vi "BC Schedule and Data Update.vi"() -> ()   [LabVIEW 2019]
doc: "This example program configures Card Number 0 as a Bus Controller\nto transmit a schedule of three messages. The schedule is\ncreated in such a way that the messages are transmitted at\nfrequencies of 100Hz, 50Hz and 25Hz (or every 10ms, 20ms and\n40ms, respectively).\n\nThe program watches the 'HIT' bit associated with the 0843H\nBC->RT message. When the message is transmitted and the\nbit is set, the program updates the data words."
uses:
  <instrlib>/BTICardLib/Private/Initialize By Card Number and Core Number.vi
  <instrlib>/BTI1553Lib/Private/Channel/Configure/Configure Channel From XML.vi
  <instrlib>/BTICardLib/BTICardLV.lvlib
  <instrlib>/BTI1553Lib/BTI1553LV.lvlib
panel:
  out "core number":i32
  out "channel number":i32
  out "Data":u16[](array[numeric]) format="%04x"
  in  "Configuration Filename":string="BCScheduleDataUpdate.FINF"
  in  "stop":bool
  out "error out":errorcluster
  in  "Card Number":i32
  # "LabVIEW RT"
  # "Mil-Std-1553: BC Schedule and Data Update"
  # "©2016 Astronics Ballard Technology"
  # "This example program configures Card Number 0 as a Bus Controller\nto transmit a schedule of three messages. The schedule is\ncreated in such a way that the messages are transmitted at\nfrequencies of 100Hz, 50Hz and 25Hz (or every 10ms, 20ms and\n40ms, respectively).\n\nThe program watches the 'HIT' bit associated with the 0843H\nBC->RT message. When the message is transmitted and the\nbit is set, the program updates the data words."
  # "LabVIEW RT can parse both XML and Binary (FINF or Fast Infoset) configuration files. While the Binary files are non-human readable, they can be loaded and parsed much more quickly than XML and are also smaller. These can also be used in LabVIEW for Windows.\n\nLabVIEW RT examples use the Binary configuration file and the corollary \"Configure From Bin\" VIs. Using the XML is as simple as switching the polymorphic configuration VI from \"Binary\" to \"XML\" and changing the Configuration Filename above."
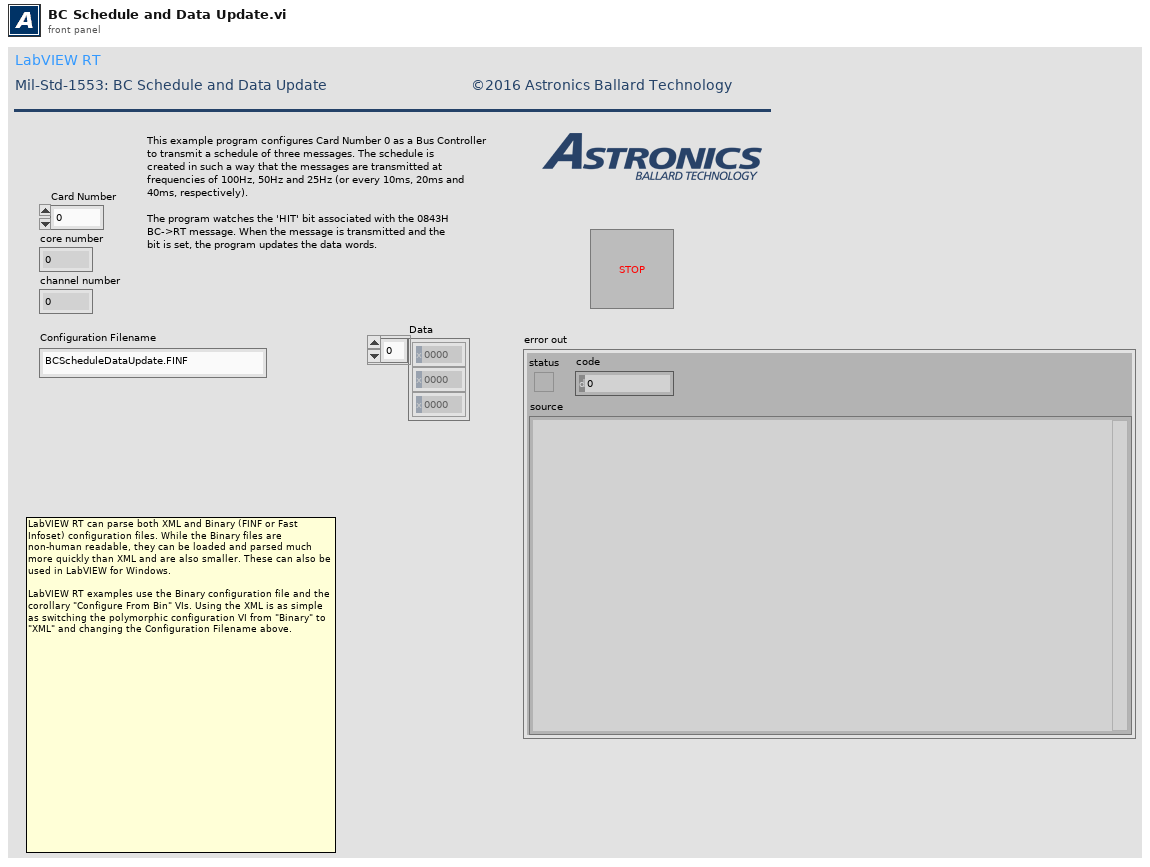
[diagram p1: front panel]
types:
  T1 = typedef "BTI1553LV.lvlib/1553 Message Fields.ctl" = cluster{"msgflag":u16, "msgopt":u16, "anyerror":bool, "noresponse":bool, "allretriesfailed":bool, "protocolerror":bool, "wrongsyncerror":bool, "datacounterror":bool, "manchestererror":bool, "parityerror":bool, "worderror":bool, "systemerror":bool, "hit":bool, "reserved":u8, "channelnumber":i32, "transmittedcwd1":bool, "transmittedcwd2":bool, "transmittedswd1":bool, "transmittedswd2":bool, "receivedcwd1":bool, "receivedcwd2":bool, "receivedswd1":bool, "receivedswd2":bool, "transmitteddwd":bool, "receiveddwd":bool, "reserved":i8, "reserved":i8, "bus":u32, "resptime1":u16, "resptime2":u16, "datacount":u16, "extflag":u16, "timetagh":u32, "timetag_hitcount":u32, "elapsetime_mintime_maxtime":u32, "cwd1":u16, "cwd2":u16, "swd1":u16, "swd2":u16, "data":u16[], "extra":u16[]}
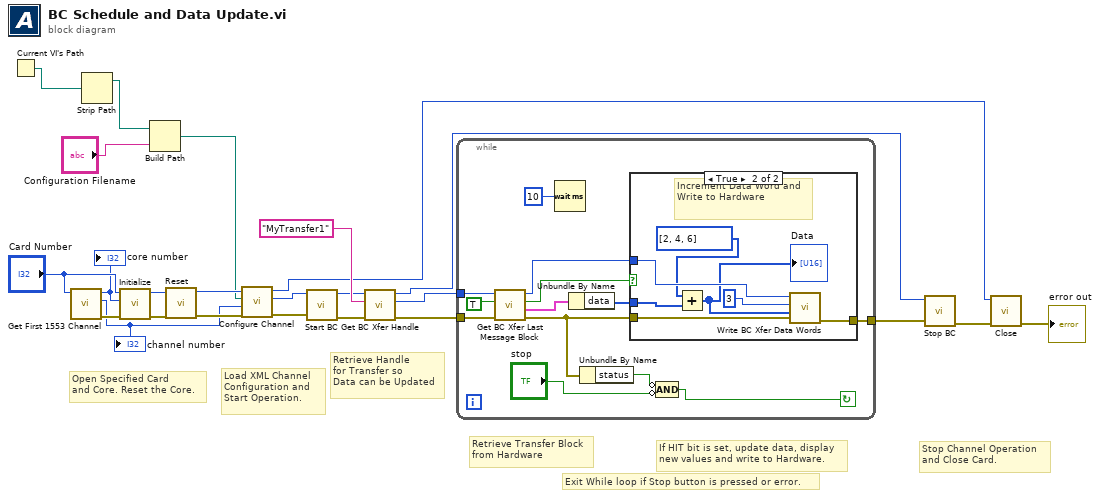
[diagram p0: block diagram]
diagram:
  # "Stop Channel Operation\nand Close Card."
  # "Exit While loop if Stop button is pressed or error."
  # "If HIT bit is set, update data, display\nnew values and write to Hardware."
  # "Retrieve Transfer Block\nfrom Hardware"
  # "Retrieve Handle\nfor Transfer so\nData can be Updated"
  # "Load XML Channel\nConfiguration and \nStart Operation."
  # "Open Specified Card\nand Core. Reset the Core."
  n1 = Current VI's Path() -> (path=w14:path)
  n2 = call "Get First 1553 Channel.vi"("Card Number"="Card Number") -> ("error out"=w4:errorcluster, "Channel Number"=w1:i32, "Core Number"=w2:i32)  [unwired: 8 in]
  "channel number" <- w1
  "core number" <- w2
  n3 = Strip Path(path=w14) -> (stripped path=w16:path)  [unwired: 1 out]
  n4 = call-poly <instrlib>:"Initialize.vi"("error in (no error)"=w4, "core number"=w2, "card number"="Card Number") -> ("error out"=w24:errorcluster, "core handle out"=w23:u64)  [unwired: 7 in]
  n5 = Build Path(base path=w16, name or relative path="Configuration Filename") -> (appended path=w15:path)
  n6 = call <instrlib>:"Reset.vi"("error in (no error)"=w24, "core handle in"=w23) -> ("error out"=w21:errorcluster, "core handle out"=w22:u64)  [unwired: 8 in]
  n7 = call-poly <instrlib>:"Configure Channel.vi"("error in (no error)"=w21, "channel number"=w1, "configuration file path"=w15, "core handle in"=w22) -> ("error out"=w19:errorcluster, "bus controller handle out"=w6:u64, "core handle out"=w8:u64)  [unwired: 1 in, 4 out]
  n8 = call <instrlib>:"Start BC.vi"("error in (no error)"=w19, "bus controller handle in"=w6) -> ("error out"=w13:errorcluster, "bus controller handle out"=w7:u64)  [unwired: 8 in]
  n9 = call <instrlib>:"Get BC Xfer Handle.vi"("error in (no error)"=w13, "bc transfer name"="MyTransfer1", "bus controller handle in"=w7) -> ("error out"=w10:errorcluster, "bc transfer handle out"=w9:u64, "bus controller handle out"=w5:u64)  [unwired: 6 in]
  n10 = while {
    tunnel: [w37] -> w11
    tunnel: w10 -> [w33]
    tunnel: w9 -> [w32]
    stop <- w36 continue-if-true
    n11 = call <instrlib>:"Get BC Xfer Last Message Block.vi"("error in (no error)"=w33, "clear hit?"=TRUE, "bc transfer handle in"=w32) -> ("error out"=w29:errorcluster, "message fields out"=w27:T1, "was hit?"=w30:bool, "bc transfer handle out"=w28:u64)  [unwired: 5 in]
    n12 = Wait (ms)(milliseconds to wait=u32 10) -> ()  [unwired: 1 out]
    n13 = Unbundle By Name(w27) -> ("data"=w26:u16[])
    n14 = Unbundle By Name(w29) -> ("status"=w34:bool)
    n15 = case shown="True" w30 {
      tunnel: w28 -> [_ w45]
      tunnel: w29 -> [w38 w43]
      tunnel: w26 -> [_ w40]
      tunnel: [w38 w42] -> w37
      frame False {
        # "Not Transmitted, So Do Nothing"
      }
      frame True {
        # "Increment Data Word and\nWrite to Hardware"
        n16 = Add(x=u16[] [2, 4, 6] ("Array"), y=w40) -> (x+y=w41:u16[])
        "Data" <- w41
        n17 = call <instrlib>:"Write BC Xfer Data Words.vi"("error in (no error)"=w43, "data words"=w41, "data word count in"=3, "bc transfer handle in"=w45) -> ("error out"=w42:errorcluster)  [unwired: 5 in, 2 out]
      }
    }
    n18 = Compound Arithmetic op=AND(invert w34, invert "stop") -> (w36:bool)
  }
  n19 = call <instrlib>:"Stop BC.vi"("error in (no error)"=w11, "bus controller handle in"=w5) -> ("error out"=w20:errorcluster)  [unwired: 8 in, 1 out]
  n20 = call <instrlib>:"Close.vi"("error in (no error)"=w20, "core handle in"=w8) -> ("error out"=→"error out":errorcluster)  [unwired: 8 in, 1 out]
